vi "Flywheel_Globals.vi"() -> ()   [LabVIEW 2019]
uses:
  Subsystems/Flywheel/Flywheel_Cluster.ctl
  Subsystems/Flywheel/Flywheel_States.ctl
panel:
  out "Flywheel_Lookup":dbl[][](array[numeric])
  out "Spun_Up":bool
  in  "Flywheel_Execute_Notifier":refnum<notifier>
  in  "Flywheel_Set_Notifier":refnum<notifier>
  in  "Flywheel_Set_Ref":string="Flywheel_Set_Ref"
  in  "Flywheel_Execute_Ref":string="Flywheel_Execute_Ref"
  in  "Flywheel_Left":string="Flywheel_Left"
  in  "Flywheel_Right":string="Flywheel_Right"
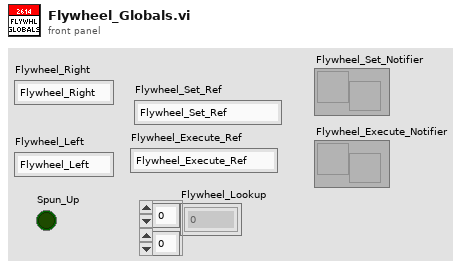
[diagram p1: front panel]
diagram:
